vi "piezoTriangleWave.vi"(1 "offset":dbl=5.0 format="%#_13g", 2 "nT":i32=1667, 3 "amplitude":dbl=1.0, 4 "omega":dbl=9.42478, 5 "t0":dbl, 6 "dt":dbl=0.00019996 format="%#_13g") -> (0 "x+y":dbl[](array[numeric]))   [LabVIEW 2017]
panel:
  out "Waveform Graph":dbl[](graph)
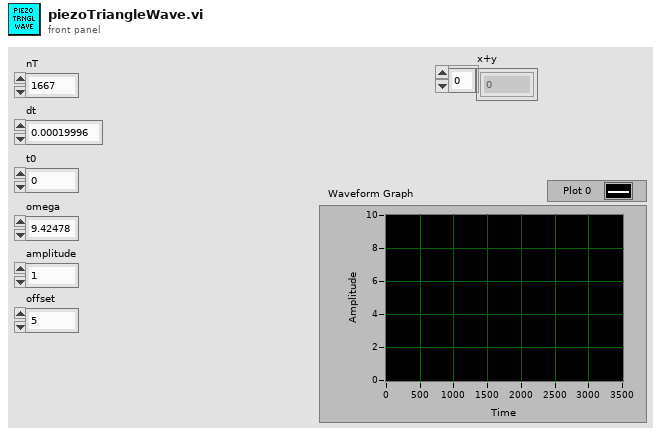
[diagram p1: front panel]
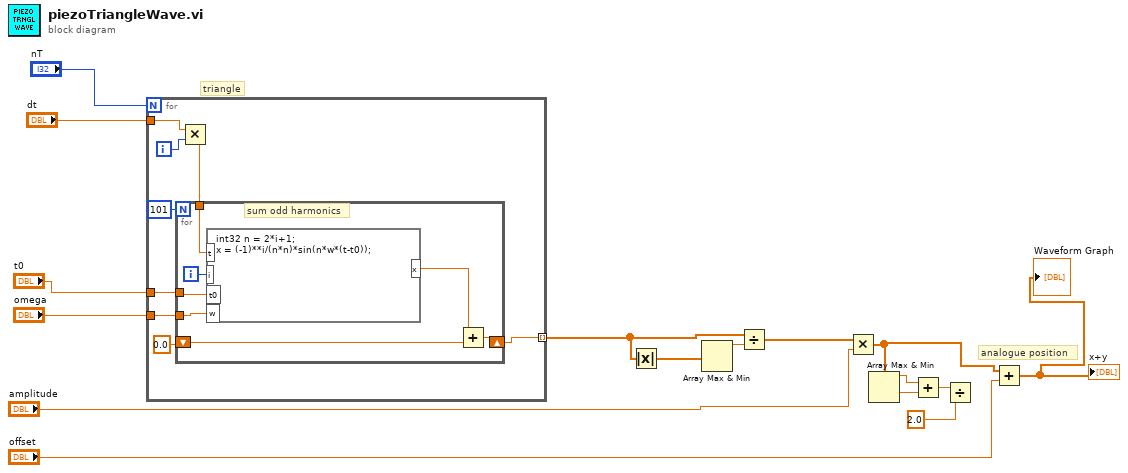
[diagram p0: block diagram]
diagram:
  # "analogue position"
  # "triangle"
  n1 = for {
    N: "nT" -> [_]
    tunnel: "dt" -> [w24]
    tunnel: "omega" -> [w21]
    tunnel: [w18] -> w8 mode=indexing
    tunnel: "t0" -> [w17]
    i -> [w23]
    n2 = Multiply(x=w24, y=w23) -> (x*y=w20:dbl)
    n3 = for {
      N: 101 -> [_]
      tunnel: w21 -> [w29]
      tunnel: w20 -> [w31]
      shift-right: [w27] -> w18
      shift-left: 0.0 -> [w26]
      tunnel: w17 -> [w25]
      i -> [w30]
      # "sum odd harmonics"
      n4 = formula code="int32 n = 2*i+1;\nx = (-1)**i/(n*n)*sin(n*w*(t-t0));"("t"=w31, "i"=w30, "w"=w29, "t0"=w25) -> ("x"=w28:dbl)
      n5 = Add(x=w28, y=w26) -> (x+y=w27:dbl)
    }
  }
  n6 = Absolute Value(x=w8) -> (abs(x)=w7:dbl[])
  n7 = Array Max & Min(array=w7) -> (max value=w6:dbl)  [unwired: 3 out]
  n8 = Divide(x=w8, y=w6) -> (x/y=w3:dbl[])
  n9 = Multiply(x=w3, y="amplitude") -> (x*y=w4:dbl[])
  n10 = Array Max & Min(array=w4) -> (max value=w14:dbl, min value=w13:dbl)  [unwired: 2 out]
  n11 = Add(x=w14, y=w13) -> (x+y=w12:dbl)
  n12 = Divide(x=w12, y=2.0) -> ()  [unwired: 1 out]
  n13 = Add(x=w4, y="offset") -> (x+y=→"x+y" →"Waveform Graph":dbl[])
